vi "Lab3.vi"() -> ()   [LabVIEW 2015]
panel:
  in  "stop":bool
  out "Boolean":bool
  in  "Numeric":dbl step=0.1
  in  "Slide":dbl(slide) scale=0.0..10.0
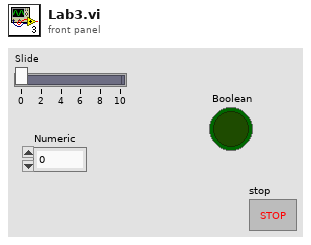
[diagram p1: front panel]
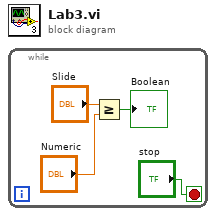
[diagram p0: block diagram]
diagram:
  n1 = while {
    stop <- "stop" stop-if-true
    n2 = Greater Or Equal?(x="Slide", y="Numeric") -> (x >= y?=→"Boolean":bool)
  }
